vi "Add Time Goal Time Stamp.vi"(10 "Time Goal (s)":dbl format="%#.6f", 11 "Starting Time (Now)":timestamp) -> (3 "Resulting Time":timestamp)   [LabVIEW 2016, in "Timer Session.lvclass"]
doc: "Calculate a future time stamp from starting time stamp and a Time Goal from Timer API."
uses:
  Timer Session.lvclass
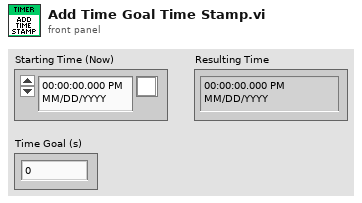
[diagram p1: front panel]
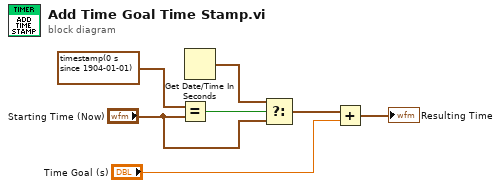
[diagram p0: block diagram]
diagram:
  n1 = Equal?(x=timestamp(0 s since 1904-01-01) ("Starting Time (Now)"), y="Starting Time (Now)") -> (x = y?=w6:bool)
  n2 = Get Date/Time In Seconds() -> (seconds since 1Jan1904=w5:timestamp)
  n3 = Select(t=w5, s=w6, f="Starting Time (Now)") -> (s? t:f=w3:timestamp)
  n4 = Add(x=w3, y="Time Goal (s)") -> (x+y=→"Resulting Time":timestamp)
